vi "LogTemp.vi"(6 "Error In (no error)":errorcluster, 8 "Path to Temp Log Folder":string="C:\\Users\\ErNa\\Documents\\LabView Codes\\ErNa Sodium Oven Controller\\Temperature Logs\\Ramp_", 9 "Temperature Log Interval (s)":dbl=10.0, 10 "Port Number":u16=2000, 11 "IP Address":string="192.168.12.200") -> (0 "Error Out":errorcluster, 2 "Temp Log Diagnosis":path=path "C:/Users/ErNa/Documents/LabView Codes/ErNa Sodium Oven Controller/Temperature Logs/Ramp_Tue, Feb 12, 2019_12-50 PM.xlsx" caption="Filename Out", 3 "Current Temperature (C)":dbl=8.0 format="%.2f")   [LabVIEW 2013, in "ovenCtrl.lvlib"]
uses:
  ovenCtrl.lvlib
panel:
  # "Inputs"
  # "Outputs"
  # "Diagnosis"
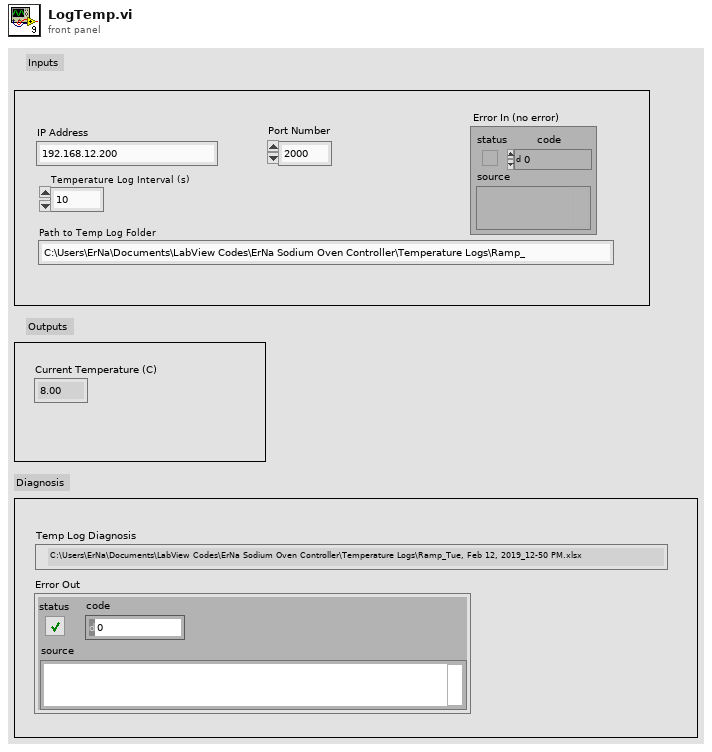
[diagram p1: front panel]
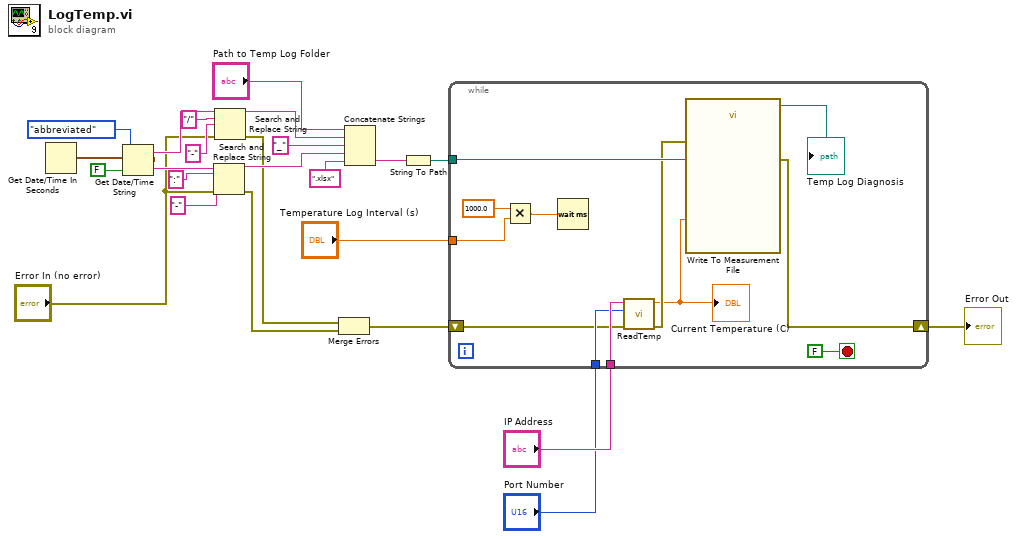
[diagram p0: block diagram]
diagram:
  n1 = Get Date/Time In Seconds() -> (seconds since 1Jan1904=w7:timestamp)
  n2 = Get Date/Time String(date format (0)=enum16{"short", "long", "abbreviated"}."abbreviated", seconds (now)=w7, want seconds? (F)=FALSE) -> (date string=w17:string, time string=w12:string)
  n3 = Search and Replace String(input string=w12, search string=":", replace string="-" ("replace string (\"\")"), error in="Error In (no error)") -> (result string=w9:string, error out=w5:errorcluster)  [unwired: 4 in, 2 out]
  n4 = Search and Replace String(input string=w17, search string="/", replace string="-" ("replace string (\"\")"), error in="Error In (no error)") -> (result string=w14:string, error out=w6:errorcluster)  [unwired: 4 in, 2 out]
  n5 = Merge Errors(w6, w5) -> (w4:errorcluster)
  n6 = Concatenate Strings("Path to Temp Log Folder", w14, "_" ("string"), w9, ".xlsx" ("string")) -> (w20:string)
  n7 = String To Path(string=w20) -> (path=w19:path)
  n8 = while {
    tunnel: "Temperature Log Interval (s)" -> [w33]
    tunnel: "IP Address" -> [w35]
    tunnel: "Port Number" -> [w34]
    tunnel: w19 -> [w31]
    shift-right: [w28] -> w1
    shift-left: w4 -> [w29]
    stop <- FALSE stop-if-true
    n9 = Multiply(x=1000.0 ("y"), y=w33) -> (x*y=w36:dbl)
    n10 = Wait (ms)(milliseconds to wait=w36) -> ()  [unwired: 1 out]
    n11 = call "ReadTemp.vi"("error in (no error)"=w29, "Port Number"=w34, "IP Address"=w35) -> ("error out"=w30:errorcluster, "Temperature"=w25:dbl)  [unwired: 7 in]
    "Current Temperature (C)" <- w25
    n12 = call "Write To Measurement File"("Signals"=w25, "error in (no error)"=w30, "Filename"=w31) -> ("Filename Out"=→"Temp Log Diagnosis":path, "error out"=w28:errorcluster)  [unwired: 14 in, 1 out]
  }
  "Error Out" <- w1
